vi "Init_Test.vi"(8 "error in (no error)":errorcluster caption="entrée d'erreur (pas d'erreur)", 11 "Wait_OpenFixture en entrée":refnum<class "Wait_OpenFixture.lvclass">) -> (0 "error out":errorcluster caption="sortie d'erreur", 3 "Wait_OpenFixture en sortie":refnum<class "Wait_OpenFixture.lvclass">)   [LabVIEW 2020, in "Library Test.lvlib" / "Wait_OpenFixture.lvclass"]
uses:
  Wait_OpenFixture.lvclass
  C:/Users/ngarcin/OneDrive - Altyor/Standard TB/Class/Test/Test (Default)/Test (Default).lvclass
  Commun VI/TypeDef/Commande Test/Commande Type Test.ctl
  Test_Without_Instr/Test_Without_Inst.lvclass
  Instrument/Instrument (Default)/Class Instrument (Default).lvclass
  Wait_OpenFixture.lvclass/Wait_OpenFixture.ctl
  Commun VI/Library Commun.lvlib
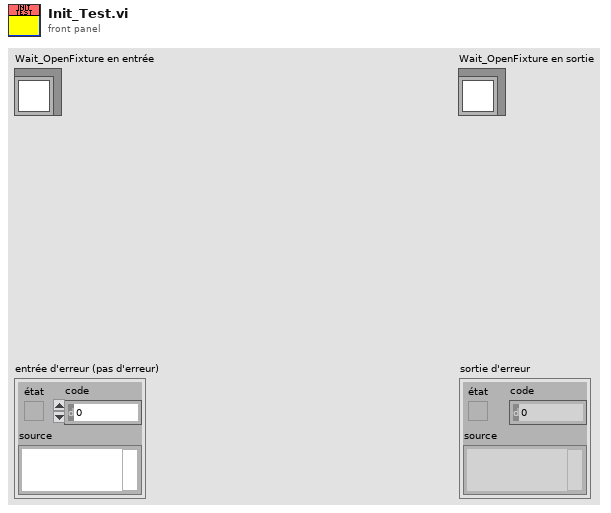
[diagram p1: front panel]
types:
  T1 = typedef "Library Commun.lvlib/Commande Type Test.ctl" = enum16{"Function", "Test", "Calculation"}
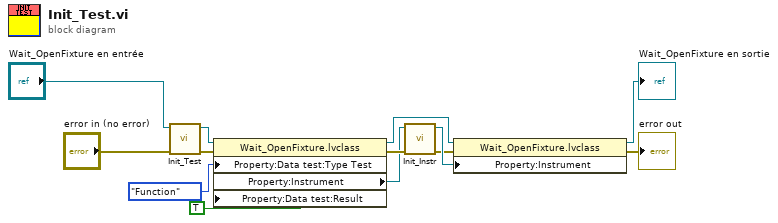
[diagram p0: block diagram]
diagram:
  n1 = call-parent "Init_Test.vi"("error in (no error)"="error in (no error)", "Test_Without_Inst en entrée"="Wait_OpenFixture en entrée") -> ("error out"=w10:errorcluster, "Test_Without_Inst en sortie"=w11:refnum<class "Wait_OpenFixture.lvclass">)  [unwired: 8 in]
  n2 = property class="Wait_OpenFixture.lvclass"(reference=w11, error in=w10, "Property:Data test:Type Test"=Commande_Type_Test."Function" ("Type Test"), "Property:Data test:Result"=TRUE ("Result")) -> (reference out=w4:refnum<class "Wait_OpenFixture.lvclass">, error out=w6:errorcluster, "Property:Instrument"=w2:refnum<class "Class Instrument (Default).lvclass">)
  n3 = call-dynamic "Init_Instr.vi"("error in (no error)"=w6, "Class Instrument (Default) en entrée"=w2) -> ("error out"=w7:errorcluster, "Class Instrument (Default) en sortie"=w8:refnum<class "Class Instrument (Default).lvclass">)  [unwired: 8 in]
  n4 = property class="Wait_OpenFixture.lvclass"(reference=w4, error in=w7, "Property:Instrument"=w8) -> (reference out=→"Wait_OpenFixture en sortie":refnum<class "Wait_OpenFixture.lvclass">, error out=→"error out":errorcluster)
